vi "Main wCredentials.vi"() -> (0 "error out":errorcluster, 3 "Weather Stations Data":T1)   [LabVIEW 2020, in "Netatmo-WeatherStation.lvlib"]
uses:
  Netatmo-WeatherStation.lvlib
  TypeDefs/body.ctl
  TypeDefs/devices.items.ctl
  TypeDefs/place.ctl
  TypeDefs/devices.dashboard_data.ctl
  TypeDefs/modules.items.ctl
  TypeDefs/modules.dashboard_data.ctl
  TypeDefs/user.ctl
  TypeDefs/administrative.ctl
  subVIs/globals.vi
panel:
  out "expire_time":timestamp
  out "Weather Stations Data (JSON)":string
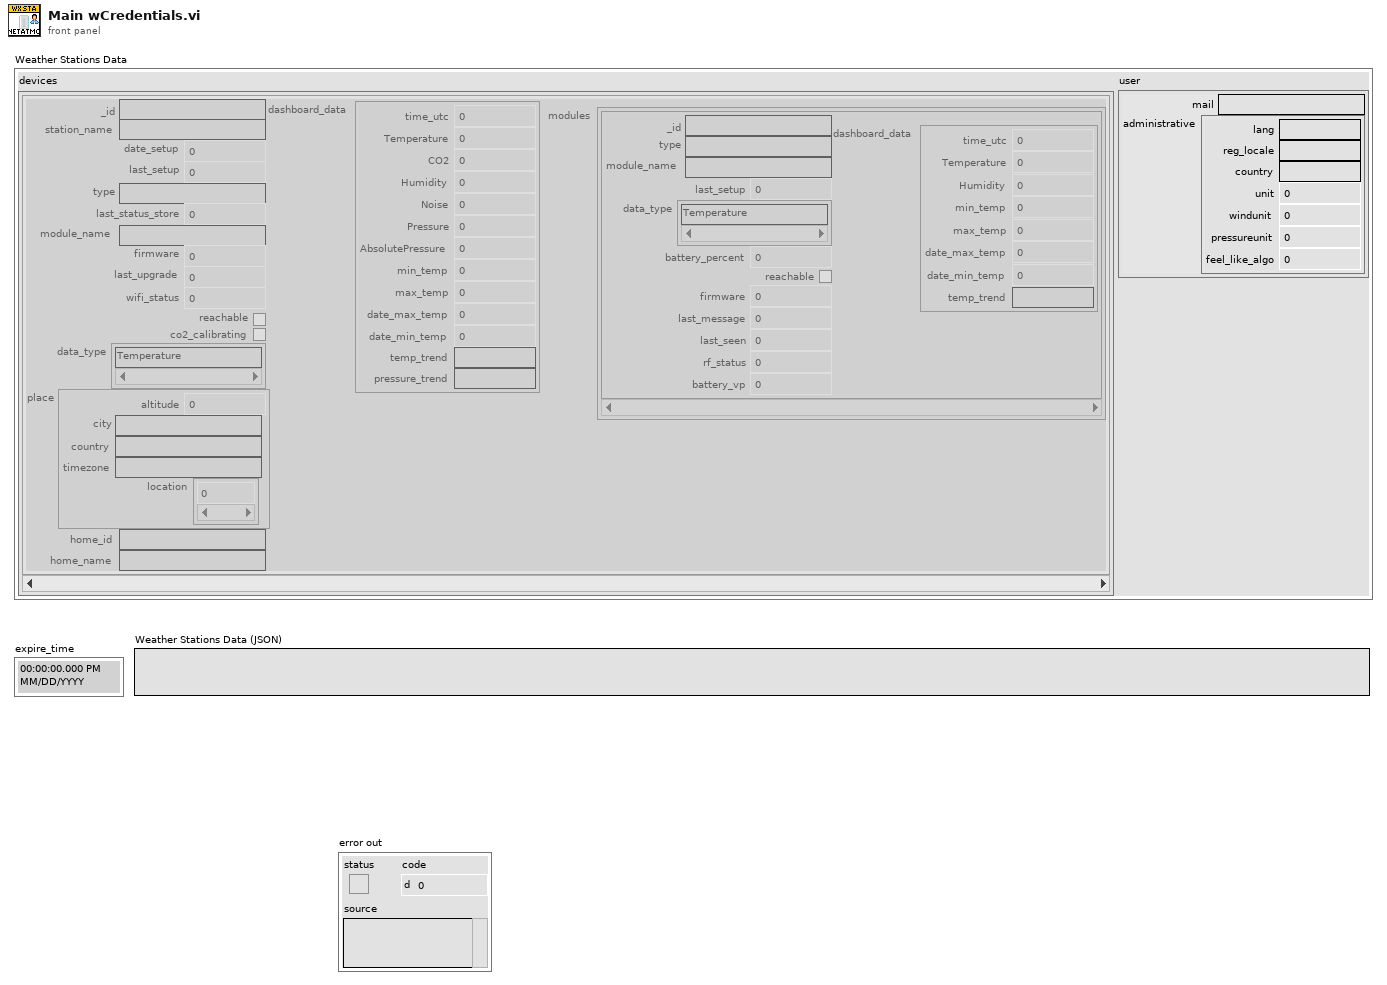
[diagram p1: front panel]
types:
  T1 = typedef "Netatmo-WeatherStation.lvlib/body.ctl" = cluster{"devices":T2[], "user":T7}
  T2 = typedef "Netatmo-WeatherStation.lvlib/devices.items.ctl" = cluster{"_id":string, "station_name":string, "date_setup":dbl, "last_setup":dbl, "type":string, "last_status_store":dbl, "module_name":string, "firmware":dbl, "last_upgrade":dbl, "wifi_status":dbl, "reachable":bool, "co2_calibrating":bool, "data_type":string[], "place":T3, "home_id":string, "home_name":string, "dashboard_data":T4, "modules":T5[]}
  T3 = typedef "Netatmo-WeatherStation.lvlib/place.ctl" = cluster{"altitude":dbl, "city":string, "country":string, "timezone":string, "location":dbl[]}
  T4 = typedef "Netatmo-WeatherStation.lvlib/devices.dashboard_data.ctl" = cluster{"time_utc":dbl, "Temperature":dbl, "CO2":dbl, "Humidity":dbl, "Noise":dbl, "Pressure":dbl, "AbsolutePressure":dbl, "min_temp":dbl, "max_temp":dbl, "date_max_temp":dbl, "date_min_temp":dbl, "temp_trend":string, "pressure_trend":string}
  T5 = typedef "Netatmo-WeatherStation.lvlib/modules.items.ctl" = cluster{"_id":string, "type":string, "module_name":string, "last_setup":dbl, "data_type":string[], "battery_percent":dbl, "reachable":bool, "firmware":dbl, "last_message":dbl, "last_seen":dbl, "rf_status":dbl, "battery_vp":dbl, "dashboard_data":T6}
  T6 = typedef "Netatmo-WeatherStation.lvlib/modules.dashboard_data.ctl" = cluster{"time_utc":dbl, "Temperature":dbl, "Humidity":dbl, "min_temp":dbl, "max_temp":dbl, "date_max_temp":dbl, "date_min_temp":dbl, "temp_trend":string}
  T7 = typedef "Netatmo-WeatherStation.lvlib/user.ctl" = cluster{"mail":string, "administrative":T8}
  T8 = typedef "Netatmo-WeatherStation.lvlib/administrative.ctl" = cluster{"lang":string, "reg_locale":string, "country":string, "unit":dbl, "windunit":dbl, "pressureunit":dbl, "feel_like_algo":dbl}
  T9 = cluster{"body":T1, "status":string, "time_exec":dbl, "time_server":dbl}
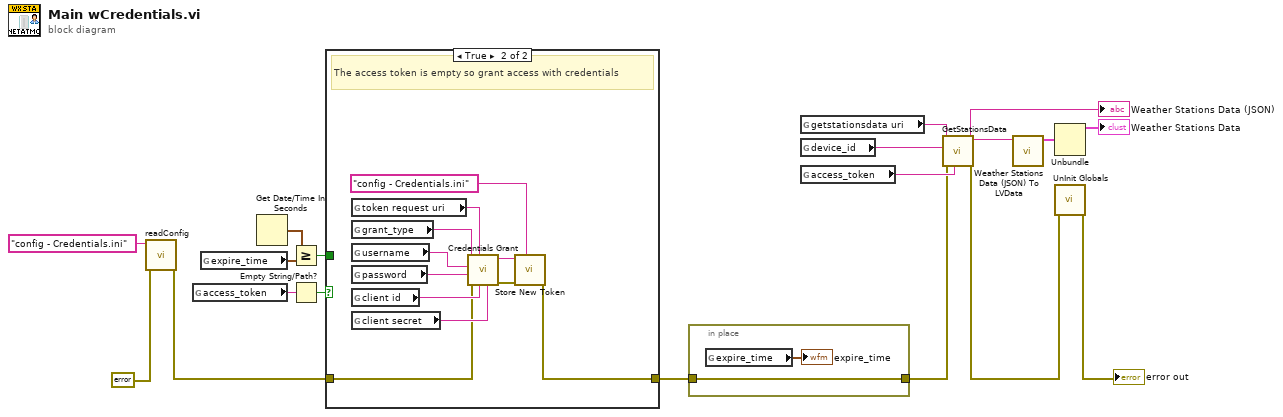
[diagram p0: block diagram]
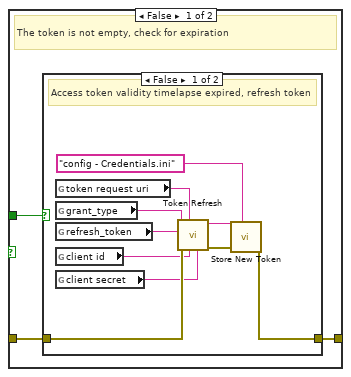
[diagram p2: hidden frame]
diagram:
  n1 = call "readConfig.vi"("error in (no error)"=errorcluster {"status"=FALSE, "code"=0, "source"=""}, "Config File Name"="config - Credentials.ini") -> ("error out"=w11:errorcluster)  [unwired: 9 in]
  n2 = global read "globals.vi" "access_token"() -> (w8:string)
  n3 = global read "globals.vi" "expire_time"() -> (w9:timestamp)
  n4 = Get Date/Time In Seconds() -> (seconds since 1Jan1904=w10:timestamp)
  n5 = Greater Or Equal?(x=w10, y=w9) -> (x >= y?=w6:bool)
  n6 = Empty String/Path?(string/path=w8) -> (empty?=w5:bool)
  n7 = case shown="True" w5 {
    tunnel: w11 -> [w21 w34]
    tunnel: [w20 w33] -> w3
    tunnel: w6 -> [w19 _]
    frame False {
      # "The token is not empty, check for expiration"
      n8 = case shown="False" w19 {
        tunnel: w21 -> [w31 w32]
        tunnel: [w23 w32] -> w20
        frame False {
          # "Access token validity timelapse expired, refresh token"
          n9 = global read "globals.vi" "token request uri"() -> (w30:string)
          n10 = global read "globals.vi" "grant_type"() -> (w29:string)
          n11 = global read "globals.vi" "refresh_token"() -> (w28:string)
          n12 = global read "globals.vi" "client id"() -> (w27:string)
          n13 = global read "globals.vi" "client secret"() -> (w26:string)
          n14 = call "Token Refresh.vi"("client secret"=w26, "client id"=w27, "token request uri"=w30, "error in (no error)"=w31, "refresh_token"=w28, "grant_type"=w29) -> ("error out"=w24:errorcluster, "token response (JSON)"=w25:string)  [unwired: 4 in]
          n15 = call "Store New Token.vi"("Config File Name"="config - Credentials.ini", "error in (no error)"=w24, "token response (JSON)"=w25) -> ("error out"=w23:errorcluster)  [unwired: 8 in]
        }
        frame True {
          # "Stil valid"
        }
      }
    }
    frame True {
      # "The access token is empty so grant access with credentials"
      n16 = global read "globals.vi" "token request uri"() -> (w43:string)
      n17 = global read "globals.vi" "grant_type"() -> (w42:string)
      n18 = global read "globals.vi" "username"() -> (w41:string)
      n19 = global read "globals.vi" "password"() -> (w40:string)
      n20 = global read "globals.vi" "client id"() -> (w39:string)
      n21 = global read "globals.vi" "client secret"() -> (w38:string)
      n22 = call "Credentials Grant.vi"("client secret"=w38, "client id"=w39, "token request uri"=w43, "error in (no error)"=w34, "password"=w40, "username"=w41, "grant_type"=w42) -> ("error out"=w37:errorcluster, "token response (JSON)"=w36:string)  [unwired: 3 in]
      n23 = call "Store New Token.vi"("Config File Name"="config - Credentials.ini", "error in (no error)"=w37, "token response (JSON)"=w36) -> ("error out"=w33:errorcluster)  [unwired: 8 in]
    }
  }
  n24 = in-place {
    in-place-border: w3 -> [w44]
    in-place-border: [w44] -> w2
    n25 = global read "globals.vi" "expire_time"() -> (→"expire_time":timestamp)
  }
  n26 = global read "globals.vi" "getstationsdata uri"() -> (w18:string)
  n27 = global read "globals.vi" "device_id"() -> (w17:string)
  n28 = global read "globals.vi" "access_token"() -> (w4:string)
  n29 = call "GetStationsData.vi"("access token"=w4, "error in (no error)"=w2, "device_id"=w17, "token request uri"=w18) -> ("error out"=w16:errorcluster, "Weather Stations Data (JSON)"=w14:string)  [unwired: 6 in]
  "Weather Stations Data (JSON)" <- w14
  n30 = call "Weather Stations Data (JSON) To LVData.vi"("Weather Stations Data (JSON)"=w14) -> ("Data"=w13:T9)  [unwired: 9 in, 1 out]
  n31 = Unbundle(w13) -> ("body"=→"Weather Stations Data":T1)  [unwired: 3 out]
  n32 = call "UnInit Globals.vi"("error in"=w16) -> ("error out"=→"error out":errorcluster)  [unwired: 10 in]
